vi "ACTIVIDAD CON INSTRUMENTOS DE MEDICION 1.vi"() -> ()   [LabVIEW 2020]
panel:
  out "subarray 2":bool[](array[boolean])
  out "s? t:f":i32
  out "subarray":bool[](array[boolean])
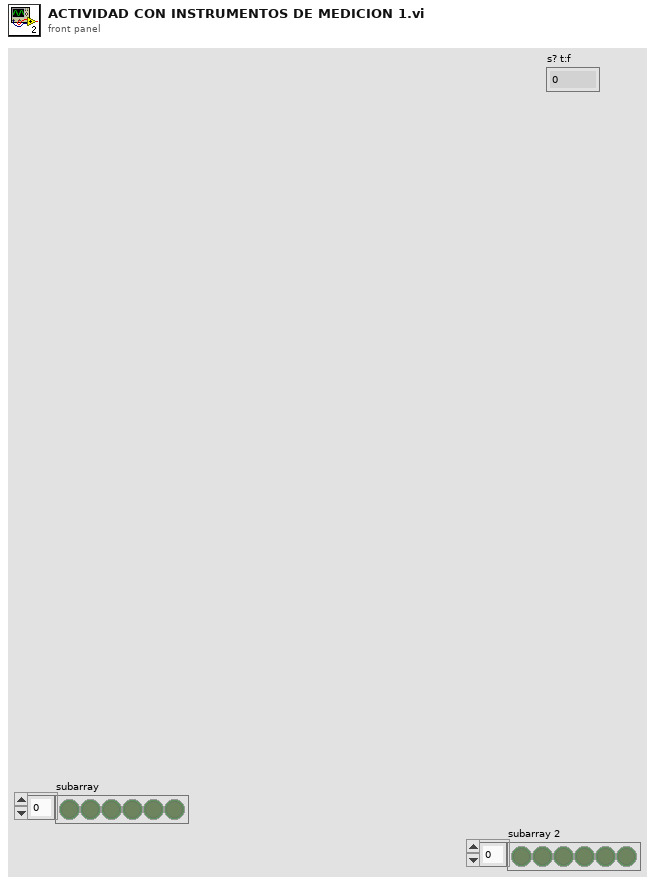
[diagram p1: front panel]
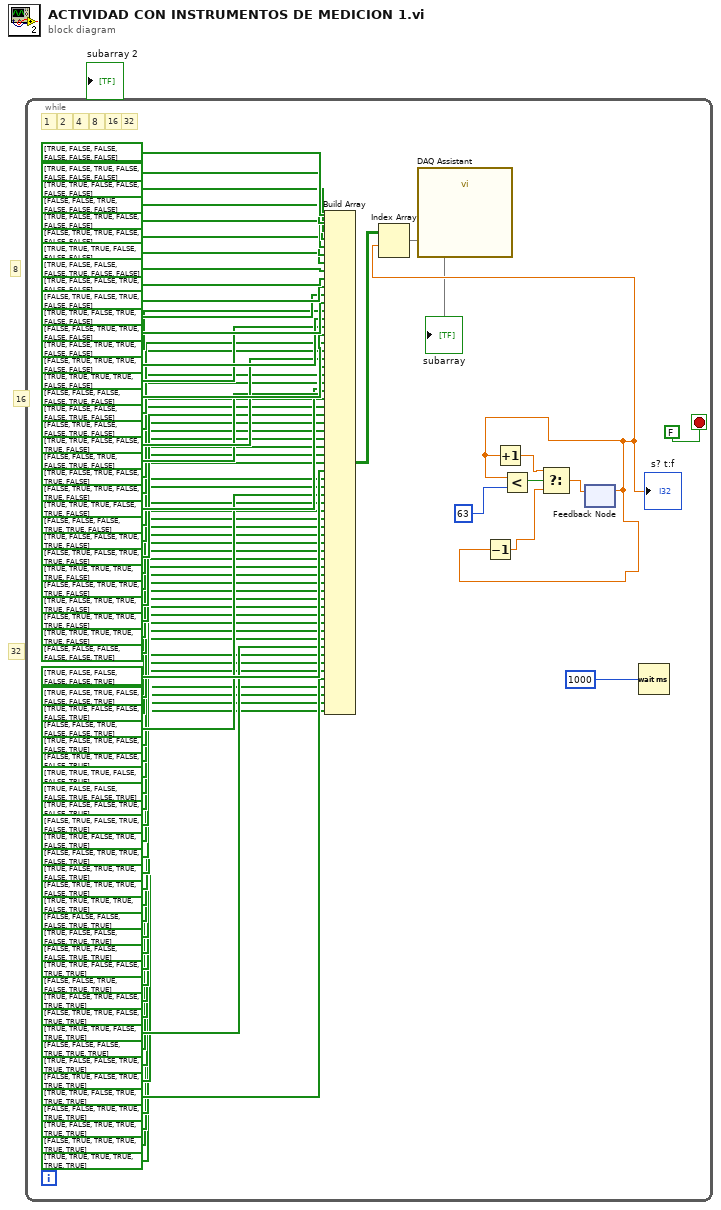
[diagram p0: block diagram]
diagram:
  # "32"
  # "16"
  # "8"
  n1 = while {
    stop <- FALSE stop-if-true
    # "32"
    # "16"
    # "8"
    # "4"
    # "2"
    # "1"
    n2 = Build Array(bool[] [TRUE, FALSE, FALSE, FALSE, FALSE, FALSE] ("#1"), bool[] [TRUE, FALSE, TRUE, FALSE, FALSE, FALSE, FALSE] ("#2"), bool[] [TRUE, TRUE, FALSE, FALSE, FALSE, FALSE] ("#3"), bool[] [FALSE, FALSE, TRUE, FALSE, FALSE, FALSE] ("#4"), bool[] [TRUE, FALSE, TRUE, FALSE, FALSE, FALSE] ("#5"), bool[] [FALSE, TRUE, TRUE, FALSE, FALSE, FALSE] ("#1"), bool[] [TRUE, TRUE, TRUE, FALSE, FALSE, FALSE] ("#3"), bool[] [TRUE, FALSE, FALSE, FALSE, TRUE, FALSE, FALSE] ("#2"), bool[] [TRUE, FALSE, FALSE, TRUE, FALSE, FALSE] ("#5"), bool[] [FALSE, TRUE, FALSE, TRUE, FALSE, FALSE] ("#4"), bool[] [TRUE, TRUE, FALSE, TRUE, FALSE, FALSE] ("#4"), bool[] [FALSE, FALSE, TRUE, TRUE, FALSE, FALSE] ("#4"), bool[] [TRUE, FALSE, TRUE, TRUE, FALSE, FALSE] ("#4"), bool[] [FALSE, TRUE, TRUE, TRUE, FALSE, FALSE] ("#4"), bool[] [TRUE, TRUE, TRUE, TRUE, FALSE, FALSE] ("#4"), bool[] [FALSE, FALSE, FALSE, FALSE, TRUE, FALSE] ("#4"), bool[] [TRUE, FALSE, FALSE, FALSE, TRUE, FALSE] ("#4"), bool[] [FALSE, TRUE, FALSE, FALSE, TRUE, FALSE] ("#4"), bool[] [TRUE, TRUE, FALSE, FALSE, TRUE, FALSE] ("#4"), bool[] [FALSE, FALSE, TRUE, FALSE, TRUE, FALSE] ("#4"), bool[] [TRUE, FALSE, TRUE, FALSE, TRUE, FALSE] ("#4"), bool[] [FALSE, TRUE, TRUE, FALSE, TRUE, FALSE] ("#4"), bool[] [TRUE, TRUE, TRUE, FALSE, TRUE, FALSE] ("#4"), bool[] [FALSE, FALSE, FALSE, TRUE, TRUE, FALSE] ("#4"), bool[] [TRUE, FALSE, FALSE, TRUE, TRUE, FALSE] ("#4"), bool[] [FALSE, TRUE, FALSE, TRUE, TRUE, FALSE] ("#4"), bool[] [TRUE, TRUE, TRUE, TRUE, TRUE, FALSE] ("#4"), bool[] [FALSE, FALSE, TRUE, TRUE, TRUE, FALSE] ("#4"), bool[] [TRUE, FALSE, TRUE, TRUE, TRUE, FALSE] ("#4"), bool[] [FALSE, TRUE, TRUE, TRUE, TRUE, FALSE] ("#4"), bool[] [TRUE, TRUE, TRUE, TRUE, TRUE, FALSE] ("#4"), bool[] [FALSE, FALSE, FALSE, FALSE, FALSE, TRUE] ("#4"), bool[] [TRUE, FALSE, FALSE, FALSE, FALSE, TRUE] ("#1"), bool[] [TRUE, FALSE, TRUE, FALSE, FALSE, FALSE, TRUE] ("#2"), bool[] [TRUE, TRUE, FALSE, FALSE, FALSE, TRUE] ("#3"), bool[] [FALSE, FALSE, TRUE, FALSE, FALSE, TRUE] ("#4"), bool[] [TRUE, FALSE, TRUE, FALSE, FALSE, TRUE] ("#5"), bool[] [FALSE, TRUE, TRUE, FALSE, FALSE, TRUE] ("#1"), bool[] [TRUE, TRUE, TRUE, FALSE, FALSE, TRUE] ("#3"), bool[] [TRUE, FALSE, FALSE, FALSE, TRUE, FALSE, TRUE] ("#2"), bool[] [TRUE, FALSE, FALSE, TRUE, FALSE, TRUE] ("#5"), bool[] [FALSE, TRUE, FALSE, TRUE, FALSE, TRUE] ("#4"), bool[] [TRUE, TRUE, FALSE, TRUE, FALSE, TRUE] ("#4"), bool[] [FALSE, FALSE, TRUE, TRUE, FALSE, TRUE] ("#4"), bool[] [TRUE, FALSE, TRUE, TRUE, FALSE, TRUE] ("#4"), bool[] [FALSE, TRUE, TRUE, TRUE, FALSE, TRUE] ("#4"), bool[] [TRUE, TRUE, TRUE, TRUE, FALSE, TRUE] ("#4"), bool[] [FALSE, FALSE, FALSE, FALSE, TRUE, TRUE] ("#4"), bool[] [TRUE, FALSE, FALSE, FALSE, TRUE, TRUE] ("#4"), bool[] [FALSE, TRUE, FALSE, FALSE, TRUE, TRUE] ("#4"), bool[] [TRUE, TRUE, FALSE, FALSE, TRUE, TRUE] ("#4"), bool[] [FALSE, FALSE, TRUE, FALSE, TRUE, TRUE] ("#4"), bool[] [TRUE, FALSE, TRUE, FALSE, TRUE, TRUE] ("#4"), bool[] [FALSE, TRUE, TRUE, FALSE, TRUE, TRUE] ("#4"), bool[] [TRUE, TRUE, TRUE, FALSE, TRUE, TRUE] ("#4"), bool[] [FALSE, FALSE, FALSE, TRUE, TRUE, TRUE] ("#4"), bool[] [TRUE, FALSE, FALSE, TRUE, TRUE, TRUE] ("#4"), bool[] [FALSE, TRUE, FALSE, TRUE, TRUE, TRUE] ("#4"), bool[] [TRUE, TRUE, FALSE, TRUE, TRUE, TRUE] ("#4"), bool[] [FALSE, FALSE, TRUE, TRUE, TRUE, TRUE] ("#4"), bool[] [TRUE, FALSE, TRUE, TRUE, TRUE, TRUE] ("#4"), bool[] [FALSE, TRUE, TRUE, TRUE, TRUE, TRUE] ("#4"), bool[] [TRUE, TRUE, TRUE, TRUE, TRUE, TRUE] ("#4")) -> (w73:bool[][])
    n3 = feedback #1() -> (w55:dbl)  [unwired: 1 in]
    "s? t:f" <- w55
    n4 = Index Array(array=w73, index (row)=w55) -> (element=w1:bool[])  [unwired: 1 in]
    "subarray" <- w1
    n5 = call "DAQ Assistant"("data"=w1) -> ()  [unwired: 17 in, 2 out]
    n6 = Decrement(x=w55) -> (x-1=w58:dbl)
    n7 = Increment(x=w55) -> (x+1=w60:dbl)
    n8 = Less?(x=w55, y=63 ("x")) -> (x < y?=w59:bool)
    n9 = Select(t=w60, s=w59, f=w58) -> (s? t:f=w57:dbl)
    n10 = feedback-in #1(w57) -> ()
    n11 = Wait (ms)(milliseconds to wait=u32 1000) -> ()  [unwired: 1 out]
  }
